vi "Settings UI.vi"() -> ()   [LabVIEW 2020, in "Performance Monitor UI.lvlib" / "Configuration.lvlib"]
doc: "Module UI that appears in the DCFG Framework for the Settings View.\n_____\nBased on DCFG Project Template 1.0.0.21.\n____\nPeloton Config 1.0.0.2\nCopyright (c) 2022, Peloton"
uses:
  Configuration.lvlib
  <vilib>/Delacor/Delacor QMH/Libraries/Cloneable Module Admin_class/Delacor_lib_QMH_Cloneable Module Admin.lvclass
  Configuration--cluster.ctl
  <vilib>/Peloton/Peloton Config/Libraries/DCFG Page/Peloton_DCFG Page.lvlib
  <vilib>/Peloton/Pelobuttons/Pelobuttons_lib_Pelobuttons.lvlib
panel:
  in  "Launch Tool":bool
  in  "Random Path":path caption="Path"
  in  "Module Admin":refnum<class "Delacor_lib_QMH_Cloneable Module Admin.lvclass">
  in  "Values in":variant
  in  "Initialized":refnum<notifier>
  # "Note: Remember to use Pelobuttons for your UI"
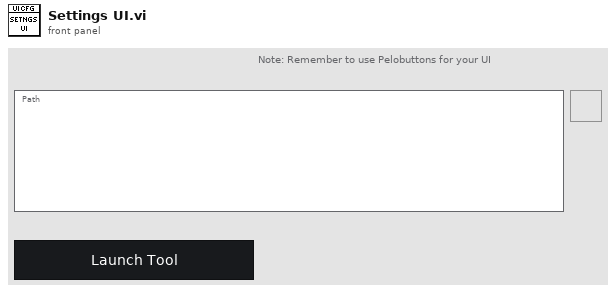
[diagram p1: front panel]
types:
  T1 = typedef "Performance Monitor UI.lvlib/Configuration.lvlib/Configuration--cluster.ctl" = cluster{"Random Path":path}
  T2 = enum32{"Invalid", "Standard", "Closed", "Hidden", "Minimized", "Maximized"}
  T3 = typedef "Peloton_DCFG Page.lvlib/Broadcast Events--cluster.ctl" = cluster{"Module Did Init":refnum<user-event>, "Status Updated":refnum<user-event>, "Error Reported":refnum<user-event>, "Module Did Stop":refnum<user-event>, "Send Data":refnum<user-event>, "Receive Data":refnum<user-event>, "Defaults Set":refnum<user-event>, "Update Module Execution Status":refnum<user-event>, "Unapplied Changes":refnum<user-event>}
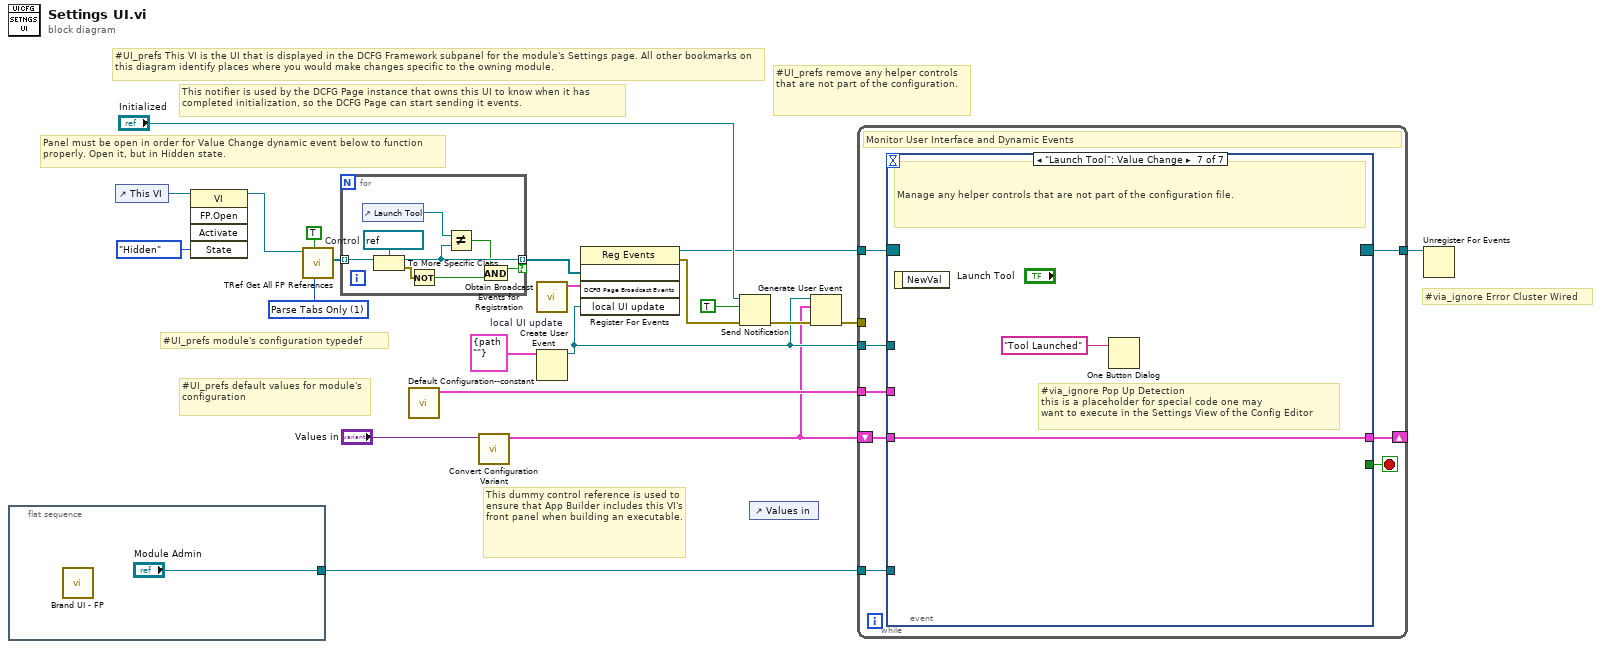
[diagram p0: block diagram]
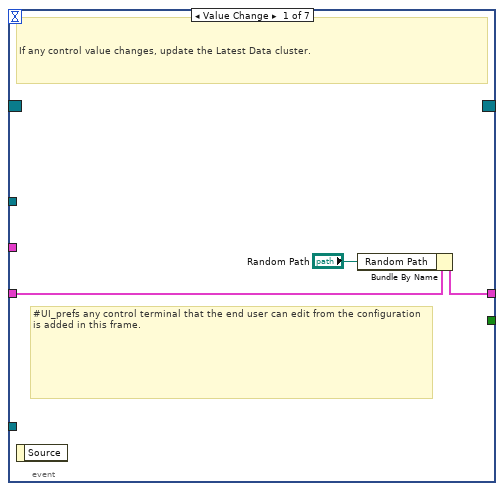
[diagram p2: hidden frame]
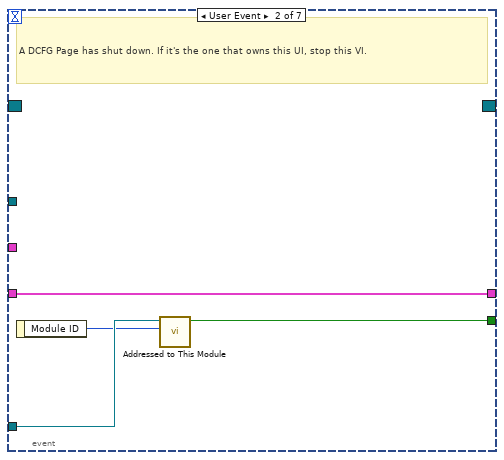
[diagram p3: hidden frame]
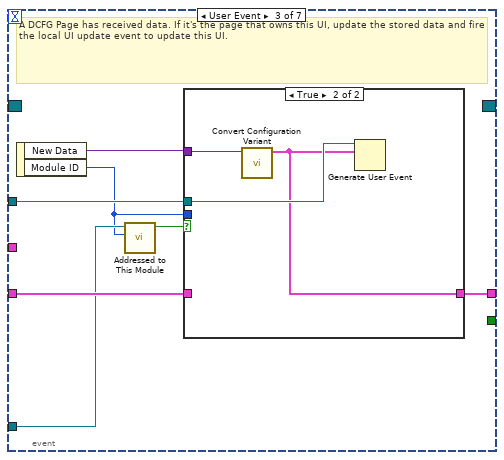
[diagram p4: hidden frame]
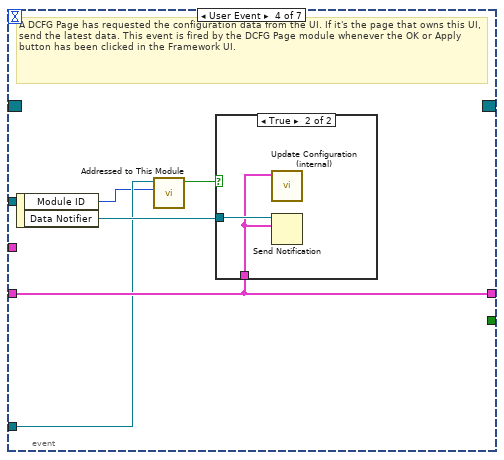
[diagram p6: hidden frame]
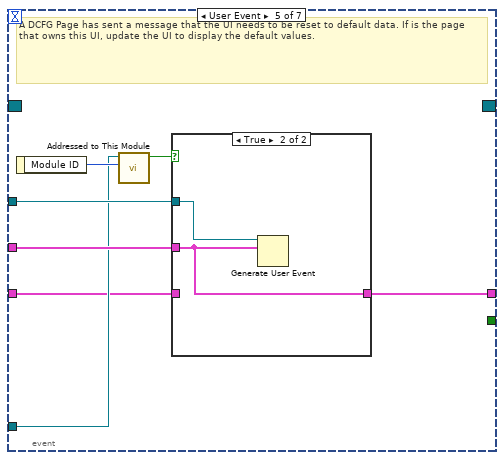
[diagram p8: hidden frame]
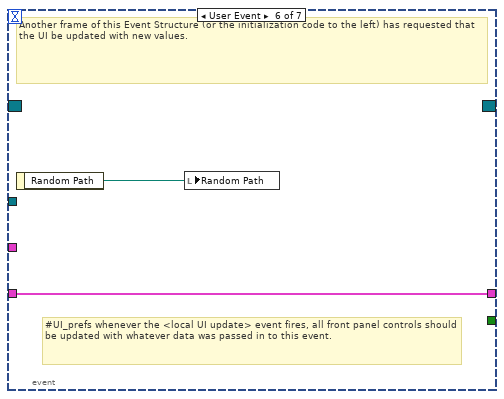
[diagram p10: hidden frame]
diagram:
  w5 = u16 1 items=["Parse All", "Parse Tabs Only"] ("Parsing Rule")
  w12 = T1 {"Random Path"=path ""}  # local UI update
  # "#via_ignore Error Cluster Wired"
  # "This dummy control reference is used to ensure that App Builder includes this VI's front panel when building an executable."
  # "#UI_prefs remove any helper controls that are not part of the configuration."
  # "Panel must be open in order for Value Change dynamic event below to function properly. Open it, but in Hidden state."
  # "This notifier is used by the DCFG Page instance that owns this UI to know when it has completed initialization, so the DCFG Page can start sending it events."
  # "#UI_prefs module's configuration typedef"
  # "#UI_prefs default values for module's configuration"
  # "#UI_prefs This VI is the UI that is displayed in the DCFG Framework subpanel for the module's Settings page. All other bookmarks on this diagram identify places where you would make changes specific to the owning module."
  n1 = flat-sequence {
    tunnel: ["Module Admin"] -> w13
    frame #0 {
      n2 = call <vilib>:"Brand UI - FP.vi"() -> ()  [unwired: 12 in]
    }
  }
  n3 = control-ref of="This VI"() -> (w1:refnum<vi>)
  n4 = invoke class="VI" method="FP.Open"(reference=w1, "State"=T2."Hidden") -> (reference out=w3:refnum<vi>)  [unwired: 3 in, 4 out]
  n5 = call <vilib>:"TRef Get All FP References.vi"("Parsing Rule"=w5, "Ignore Decorations?"=TRUE, "VI Refnum"=w3) -> ("All FP Objects"=w4:refnum<vi>[])  [unwired: 4 in, 4 out]
  n6 = for {
    tunnel: w4 -> [w30] mode=indexing
    tunnel: [w25] -> w2 mode=indexing if=w26
    w29 = refnum<vi> refnum  # Control
    n7 = control-ref of="Launch Tool"() -> (w23:refnum<vi>)
    n8 = To More Specific Class(target class=w29, reference=w30) -> (specific class reference=w25:refnum<vi>, error out=w28:errorcluster)  [unwired: 1 in]
    n9 = Not(x=w28) -> (.not. x?=w27:bool)
    n10 = Not Equal?(x=w23, y=w25) -> (x != y?=w24:bool)
    n11 = And(x=w24, y=w27) -> (x .and. y?=w26:bool)
  }
  n12 = call "Default Configuration--constant.vi"() -> ("Default Configuration"=w9:T1)  [unwired: 11 in]
  n13 = call "Convert Configuration Variant.vi"("Current Configuration"="Values in") -> ("Configuration"=w8:T1)  [unwired: 8 in, 2 out]
  n14 = call <vilib>:"Obtain Broadcast Events for Registration.vi"() -> ("DCFG Page Broadcast Events"=w20:T3)  [unwired: 9 in, 2 out]
  n15 = Create User Event(user event datatype=w12) -> (user event=w10:refnum<user-event>)  [unwired: 1 in, 1 out]
  n16 = register-events(w2, w20, w10) -> (reference out=w16:refnum<event-registration>, error out=w14:errorcluster)  [unwired: 2 in]
  n17 = Send Notification(notification=TRUE, notifier="Initialized", error in (no error)=w14) -> (error out=w17:errorcluster)  [unwired: 1 out]
  n18 = control-ref of="Values in"() -> ()  [unwired: 1 out]
  n19 = Generate User Event(user event=w10, event data cluster=w8, error in=w17) -> (error out=w11:errorcluster)  [unwired: 1 in, 1 out]
  n20 = while {
    tunnel: w11 -> [_]
    tunnel: w16 -> [w38]
    tunnel: [w37] -> w15
    shift-right: [w33] -> _
    shift-left: w8 -> [w36]
    tunnel: w13 -> [w34]
    tunnel: w9 -> [w32]
    tunnel: w10 -> [w31]
    stop <- w35 stop-if-true
    # "Monitor User Interface and Dynamic Events"
    n21 = event shown="[6] \"Launch Tool\": Value Change" {
      selector: w38 -> [_ _ _ _ _ _ _]
      dyn-events: [_ _ _ _ _ _ _] -> w37
      timeout: _ -> [_ _ _ _ _ _ _]
      tunnel: w36 -> [w41 w45 w52 w60 w65 w75 w77]
      tunnel: [w40 w45 w51 w60 w64 w75 w77] -> w33
      tunnel: [_ w42 _ _ _ _ _] -> w35
      tunnel: w34 -> [_ w44 w47 w59 w67 _ _]
      tunnel: w32 -> [_ _ _ _ w70 _ _]
      tunnel: w31 -> [_ _ w49 _ w69 _ _]
      event Value Change {
        # "#UI_prefs any control terminal that the end user can edit from the configuration is added in this frame."
        # "If any control value changes, update the Latest Data cluster."
        n22 = event-data() -> ()  [unwired: 1 in, 1 out]
        n23 = Bundle By Name(cluster=w41, "Random Path"="Random Path") -> (w40:T1)
      }
      event User Event {
        # "A DCFG Page has shut down. If it's the one that owns this UI, stop this VI."
        n24 = event-data() -> ("Module ID"=w43:i32)  [unwired: 1 in]
        n25 = call <vilib>:"Addressed to This Module.vi"("Module ID from Argument"=w43, "Module Admin"=w44) -> ("Addressed to this instance?"=w42:bool)  [unwired: 8 in, 1 out]
      }
      event User Event {
        # "A DCFG Page has received data. If it's the page that owns this UI, update the stored data and fire the local UI update event to update this UI."
        n26 = event-data() -> ("New Data"=w50:variant, "Module ID"=w46:i32)  [unwired: 1 in]
        n27 = call <vilib>:"Addressed to This Module.vi"("Module ID from Argument"=w46, "Module Admin"=w47) -> ("Addressed to this instance?"=w48:bool)  [unwired: 8 in, 1 out]
        n28 = case shown="True" w48 {
          tunnel: w52 -> [w53 _]
          tunnel: [w53 w54] -> w51
          tunnel: w50 -> [_ w55]
          tunnel: w49 -> [_ w56]
          tunnel: w46 -> [_ _]
          frame False {
          }
          frame True {
            n29 = call "Convert Configuration Variant.vi"("Current Configuration"=w55) -> ("Configuration"=w54:T1)  [unwired: 8 in, 2 out]
            n30 = Generate User Event(user event=w56, event data cluster=w54) -> ()  [unwired: 2 in, 2 out]
          }
        }
      }
      event User Event {
        # "A DCFG Page has requested the configuration data from the UI. If it's the page that owns this UI, send the latest data. This event is fired by the DCFG Page module whenever the OK or Apply button has been clicked in the Framework UI."
        n31 = event-data() -> ("Module ID"=w57:i32, "Data Notifier"=w61:refnum<notifier>)  [unwired: 1 in]
        n32 = call <vilib>:"Addressed to This Module.vi"("Module ID from Argument"=w57, "Module Admin"=w59) -> ("Addressed to this instance?"=w58:bool)  [unwired: 8 in, 1 out]
        n33 = case shown="True" w58 {
          tunnel: w61 -> [_ w63]
          tunnel: w60 -> [_ w62]
          frame False {
          }
          frame True {
            n34 = call "Update Configuration (internal).vi"("configuration"=w62) -> ()  [unwired: 11 in]
            n35 = Send Notification(notification=w62, notifier=w63) -> ()  [unwired: 1 in, 2 out]
          }
        }
      }
      event User Event {
        # "A DCFG Page has sent a message that the UI needs to be reset to default data. If is the page that owns this UI, update the UI to display the default values."
        n36 = event-data() -> ("Module ID"=w68:i32)  [unwired: 1 in]
        n37 = call <vilib>:"Addressed to This Module.vi"("Module ID from Argument"=w68, "Module Admin"=w67) -> ("Addressed to this instance?"=w66:bool)  [unwired: 8 in, 1 out]
        n38 = case shown="True" w66 {
          tunnel: w70 -> [_ w72]
          tunnel: w69 -> [_ w73]
          tunnel: w65 -> [w71 _]
          tunnel: [w71 w72] -> w64
          frame False {
          }
          frame True {
            n39 = Generate User Event(user event=w73, event data cluster=w72) -> ()  [unwired: 2 in, 2 out]
          }
        }
      }
      event User Event {
        # "#UI_prefs whenever the <local UI update> event fires, all front panel controls should be updated with whatever data was passed in to this event."
        # "Another frame of this Event Structure (or the initialization code to the left) has requested that the UI be updated with new values."
        n40 = event-data() -> ("Random Path"=w74:path)  [unwired: 1 in]
        n41 = local write "Random Path"(w74) -> ()
      }
      event "Launch Tool": Value Change {
        # "#via_ignore Pop Up Detection\nthis is a placeholder for special code one may \nwant to execute in the Settings View of the Config Editor"
        # "Manage any helper controls that are not part of the configuration file."
        n42 = event-data() -> ()  [unwired: 1 in, 1 out]
        n43 = One Button Dialog(message="Tool Launched") -> ()  [unwired: 1 in, 1 out]
      }
    }
  }
  n44 = Unregister For Events(event registration refnum=w15) -> ()  [unwired: 1 in, 1 out]
